vi "test-TimeInterpBoolean-ALL-TESTS.vi"(8 "error in (no error)":errorcluster) -> (0 "error out":errorcluster, 3 "All Passed":bool)   [LabVIEW 2019]
panel:
  out "Test 1":bool
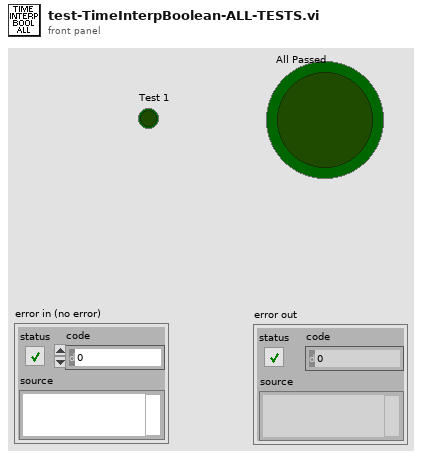
[diagram p1: front panel]
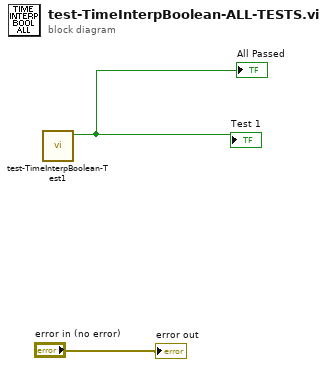
[diagram p0: block diagram]
diagram:
  n1 = call "test-TimeInterpBoolean-Test1.vi"() -> ("All tests passed"=→"All Passed" →"Test 1":bool)  [unwired: 11 in]
  "error out" <- "error in (no error)"
